vi "Initialize Root Paras.vi"(5 "Allowed VI Alias":string[](array[string]), 6 "RootQueueName":string, 7 "Allowed VI Path":path[](array[path]), 8 "error in (no error)":errorcluster caption="错误输入（无错误）", 9 "CurrentVi*":refnum<vi>, 10 "RootPanel*":refnum<vi>, 11 "PanelRootNode 输入":refnum<class "PanelRootNode.lvclass"> caption="DNL_LabVIEW Object in") -> (0 "error out":errorcluster caption="错误输出", 2 "SelfNode*":refnum<data-value>)   [LabVIEW 2016, in "PanelRootNode.lvclass"]
uses:
  PanelRootNode.lvclass
  C:/Users/CL/Desktop/ZcDAQprj0811/ZcDAQprj/Modules/DAQ-Display/PanelSplitToolkit/PanelDataNode/PanelDataNode.lvclass
  PanelRootNode.lvclass/PanelRootNode.ctl
  PanelDataNode/PanelDataNode.lvclass/PanelDataNode.ctl
  PanelDataNode/PanelDataNode.lvclass
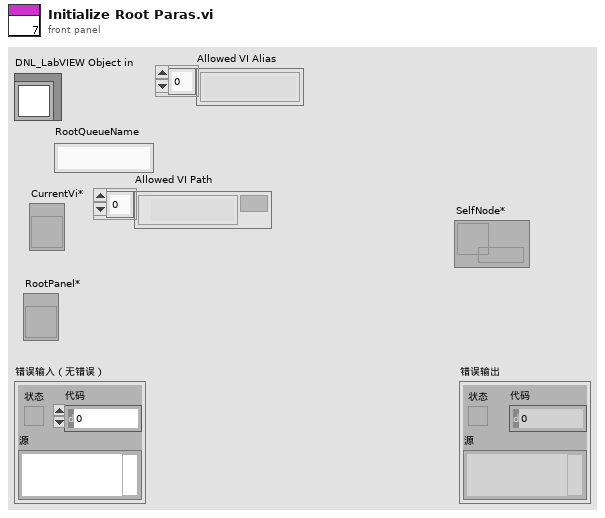
[diagram p1: front panel]
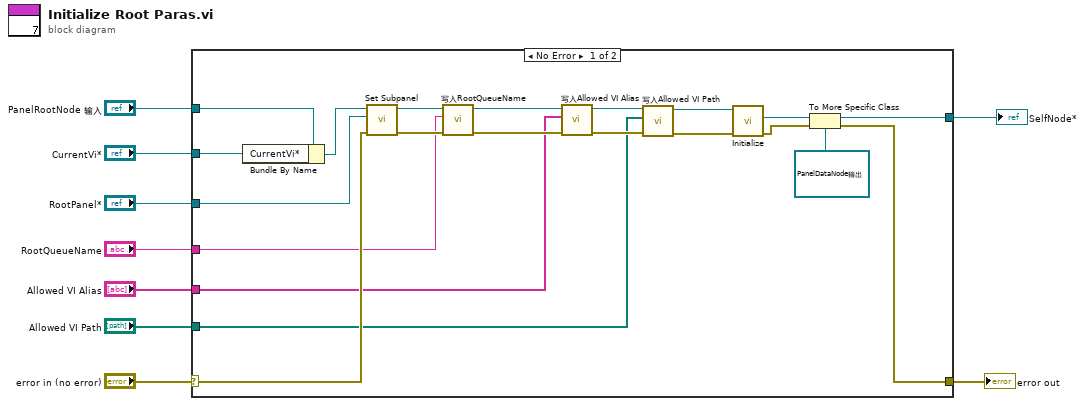
[diagram p0: block diagram]
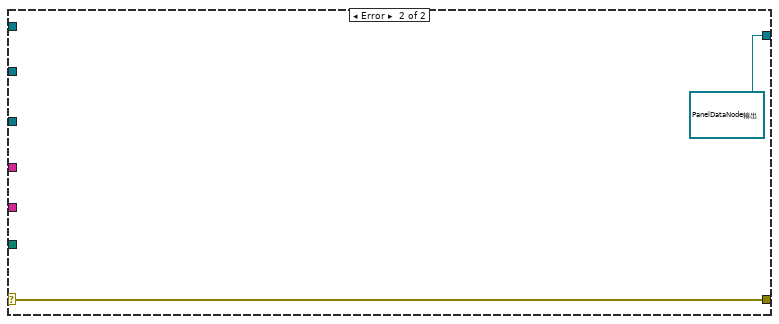
[diagram p2: hidden frame]
diagram:
  n1 = case shown="No Error" "error in (no error)" {
    selector: "error in (no error)" -> [w13 w32]
    tunnel: [w14 w32] -> w8
    tunnel: "PanelRootNode 输入" -> [w22 _]
    tunnel: "RootPanel*" -> [w30 _]
    tunnel: [w28 refnum<data-value> refnum ("data value reference")] -> w5
    tunnel: "CurrentVi*" -> [w16 _]
    tunnel: "RootQueueName" -> [w12 _]
    tunnel: "Allowed VI Alias" -> [w11 _]
    tunnel: "Allowed VI Path" -> [w10 _]
    frame No Error {
      n2 = Bundle By Name(cluster=w22, "CurrentVi*"=w16) -> (w21:refnum<class "PanelRootNode.lvclass">)
      n3 = call "Set Subpanel.vi"("error in (no error)"=w13, "Subpanel*"=w30, "PanelDataNode输入"=w21) -> ("error out"=w20:errorcluster, "PanelDataNode输出"=w19:refnum<class "PanelRootNode.lvclass">)  [unwired: 7 in]
      n4 = call "写入RootQueueName.vi"("error in (no error)"=w20, "RootQueueName"=w12, "PanelDataNode输入"=w19) -> ("error out"=w17:errorcluster, "PanelDataNode输出"=w18:refnum<class "PanelRootNode.lvclass">)  [unwired: 7 in]
      n5 = call "写入Allowed VI Alias.vi"("error in (no error)"=w17, "Allowed VI Alias"=w11, "PanelDataNode输入"=w18) -> ("error out"=w24:errorcluster, "PanelDataNode输出"=w26:refnum<class "PanelRootNode.lvclass">)  [unwired: 7 in]
      n6 = call "写入Allowed VI Path.vi"("error in (no error)"=w24, "Allowed VI Path"=w10, "PanelDataNode输入"=w26) -> ("error out"=w23:errorcluster, "PanelDataNode输出"=w25:refnum<class "PanelRootNode.lvclass">)  [unwired: 7 in]
      n7 = call-dynamic "Initialize.vi"("error in"=w23, "PanelRootNode in"=w25) -> ("error out"=w15:errorcluster, "SelfNode*"=w29:refnum<data-value>)  [unwired: 7 in]
      n8 = To More Specific Class(target class=refnum<data-value> refnum ("数据值引用"), reference=w29, error in=w15) -> (specific class reference=w28:refnum<data-value>, error out=w14:errorcluster)
    }
    frame Error {
    }
  }
  "error out" <- w8
  "SelfNode*" <- w5
